vi "gigaseal_checker.vi"(8 "default val in beginning":bool, 10 "num elements to look at":i32=3, 11 "gigasealing array":dbl[](array[numeric])) -> (3 "Gigaseal?":bool)   [LabVIEW 2015]
uses:
  <vilib>/Analysis/NI_AALBase.lvlib
  <vilib>/Analysis/baseanly.llb/Mean (DBL).vi
panel:
  in  "gigasealing array 2":dbl[](array[numeric])
  out "subarray":dbl[](array[numeric])
  # "earliest"
  # "latest"
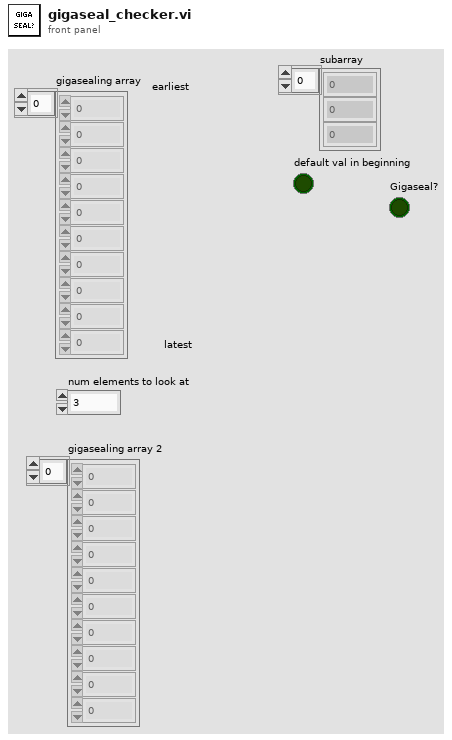
[diagram p1: front panel]
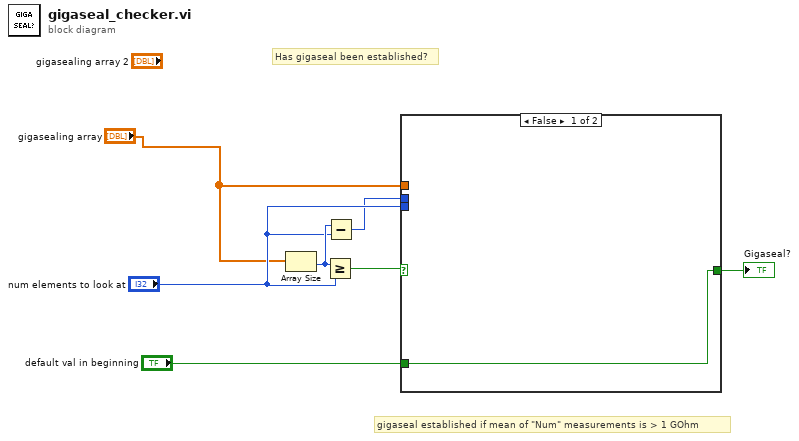
[diagram p0: block diagram]
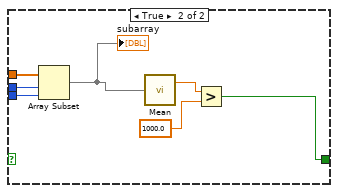
[diagram p2: hidden frame]
diagram:
  # "gigaseal established if mean of \"Num\" measurements is > 1 GOhm"
  # "Has gigaseal been established?"
  n1 = Array Size(array="gigasealing array") -> (size(s)=w7:i32)
  n2 = Greater Or Equal?(x=w7, y="num elements to look at") -> (x >= y?=w3:bool)
  n3 = Subtract(x=w7, y="num elements to look at") -> (x-y=w5:i32)
  n4 = case shown="False" w3 {
    tunnel: "num elements to look at" -> [_ w15]
    tunnel: w5 -> [_ w14]
    tunnel: "gigasealing array" -> [_ w13]
    tunnel: [w8 w9] -> w2
    tunnel: "default val in beginning" -> [w8 _]
    frame False {
    }
    frame True {
      n5 = Array Subset(array=w13, index=w14, length=w15) -> (w12:dbl[])
      "subarray" <- w12
      n6 = call-poly <vilib>:"Mean.vi"("X"=w12) -> ("mean"=w11:dbl)  [unwired: 1 out]
      n7 = Greater?(x=w11, y=1000.0) -> (0:w9:bool)
    }
  }
  "Gigaseal?" <- w2
